vi "Unit Test Parent Level Renamed.vi"() -> ()   [LabVIEW 2019, in "Sports Unit Tests.lvclass"]
uses:
  Sports Unit Tests.lvclass
  Classes/John Cena/John Cena.lvclass
  <vilib>/Utility/error.llb/Clear Errors.vi
  <vilib>/addons/_JKI Toolkits/Caraya/classes/Test/Define Test.vi
  <vilib>/addons/_JKI Toolkits/Caraya/classes/Assert/Assert Equal Value_Variant.vi
  <vilib>/addons/_JKI Toolkits/Caraya/classes/Assert/Assert Not Error.vi
  <userlib>/Blue Origin/BlueSerialization/BlueSerializer/BlueSerializer.lvclass
  <vilib>/addons/_JKI Toolkits/Caraya/classes/Assert/Assert.lvclass
panel:
  out "Table":string[][](table)=[["{\r  \"Class\":[\"John Cena.lvclass\",\"WWF Wrestler.lvclass\",\"Sports Player.lvclass\",\"Human.lvclass\",\"BlueSerialization.lvlib:BlueSerializable.lvclass\"],\r  \"Version\":[\"2.0.0.3\",\"2.0.0.3\",\"2.0.0.3\",\"2.0.0.3\",\"2.0.0.0\"],\r  \"BlueSerialization.lvlib:BlueSerializable.lvclass\":{\"LibVersion\":1},\r  \"Human.lvclass\":{\r    \"alive?\":true,\r    \"Age (years)\":40,\r    \"Name\":\"John Cena\",\r    \"Height (ft)\":6\r  },\r  \"Sports Player.lvclass\":{\r    \"Professional?\":true,\r    \"Earnings (dollars)\":1000000,\r    \"Sponsor\":\"Monster Energy\"\r  },\r  \"WWF Wrestler.lvclass\":{\r    \"Current champion?\":false,\r    \"# champion titles\":6,\r    \"Weight (lbs)\":250\r  },\r  \"John Cena.lvclass\":{\"Latest movie role\":\"The Marine\"}\r}", "{\r  \"Class\":[\"John Cena.lvclass\",\"WWF Wrestler.lvclass\",\"Sports Player.lvclass\",\"Human.lvclass\",\"BlueSerialization.lvlib:BlueSerializable.lvclass\"],\r  \"Version\":[\"2.0.0.3\",\"2.0.0.3\",\"2.0.0.3\",\"2.0.0.3\",\"2.0.0.0\"],\r  \"BlueSerialization.lvlib:BlueSerializable.lvclass\":{\"LibVersion\":1},\r  \"Human.lvclass\":{\r    \"alive?\":true,\r    \"Age (years)\":40,\r    \"Name\":\"John Cena\",\r    \"Height (ft)\":6\r  },\r  \"Sports Player.lvclass\":{\r    \"Professional?\":true,\r    \"Earnings (dollars)\":1000000,\r    \"Sponsor\":\"Monster Energy\"\r  },\r  \"WWF Wrestler.lvclass\":{\r    \"Current champion?\":false,\r    \"# champion titles\":6,\r    \"Weight (lbs)\":250\r  },\r  \"John Cena.lvclass\":{\"Latest movie role\":\"The Marine\"}\r}", "Status: FALSE\ncode: 0\n", "BlueJSONTextSerializer.lvlib:BlueJSONTextSerializer.lvclass"], ["Class = [\"John Cena.lvclass\", \"WWF Wrestler.lvclass\", \"Sports Player.lvclass\", \"Human.lvclass\", \"BlueSerialization.lvlib:BlueSerializable.lvclass\"]\r\nVersion = [\"2.0.0.3\", \"2.0.0.3\", \"2.0.0.3\", \"2.0.0.3\", \"2.0.0.0\"]\r\n\n[\"BlueSerialization.lvlib:BlueSerializable.lvclass\"]\nLibVersion = 1\r\n\n[\"Human.lvclass\"]\n\"alive?\" = true\r\n\"Age (years)\" = 40\r\nName = \"John Cena\"\r\n\"Height (ft)\" = 6.0\r\n\n[\"Sports Player.lvclass\"]\n\"Professional?\" = true\r\n\"Earnings (dollars)\" = 1000000.0\r\nSponsor = \"Monster Energy\"\r\n\n[\"WWF Wrestler.lvclass\"]\n\"Current champion?\" = false\r\n\"# champion titles\" = 6\r\n\"Weight (lbs)\" = 250.0\r\n\n[\"John Cena.lvclass\"]\n\"Latest movie role\" = \"The Marine\"\r\n", "Class = [\"John Cena.lvclass\", \"WWF Wrestler.lvclass\", \"Sports Player.lvclass\", \"Human.lvclass\", \"BlueSerialization.lvlib:BlueSerializable.lvclass\"]\r\nVersion = [\"2.0.0.3\", \"2.0.0.3\", \"2.0.0.3\", \"2.0.0.3\", \"2.0.0.0\"]\r\n\n[\"BlueSerialization.lvlib:BlueSerializable.lvclass\"]\nLibVersion = 1\r\n\n[\"Human.lvclass\"]\n\"alive?\" = true\r\n\"Age (years)\" = 40\r\nName = \"John Cena\"\r\n\"Height (ft)\" = 6.0\r\n\n[\"Sports Player.lvclass\"]\n\"Professional?\" = true\r\n\"Earnings (dollars)\" = 1000000.0\r\nSponsor = \"Monster Energy\"\r\n\n[\"WWF Wrestler.lvclass\"]\n\"Current champion?\" = false\r\n\"# champion titles\" = 6\r\n\"Weight (lbs)\" = 250.0\r\n\n[\"John Cena.lvclass\"]\n\"Latest movie role\" = \"The Marine\"\r\n", "Status: FALSE\ncode: 0\n", "BlueTOMLSerializer.lvlib:BlueTOMLSerializer.lvclass"]]
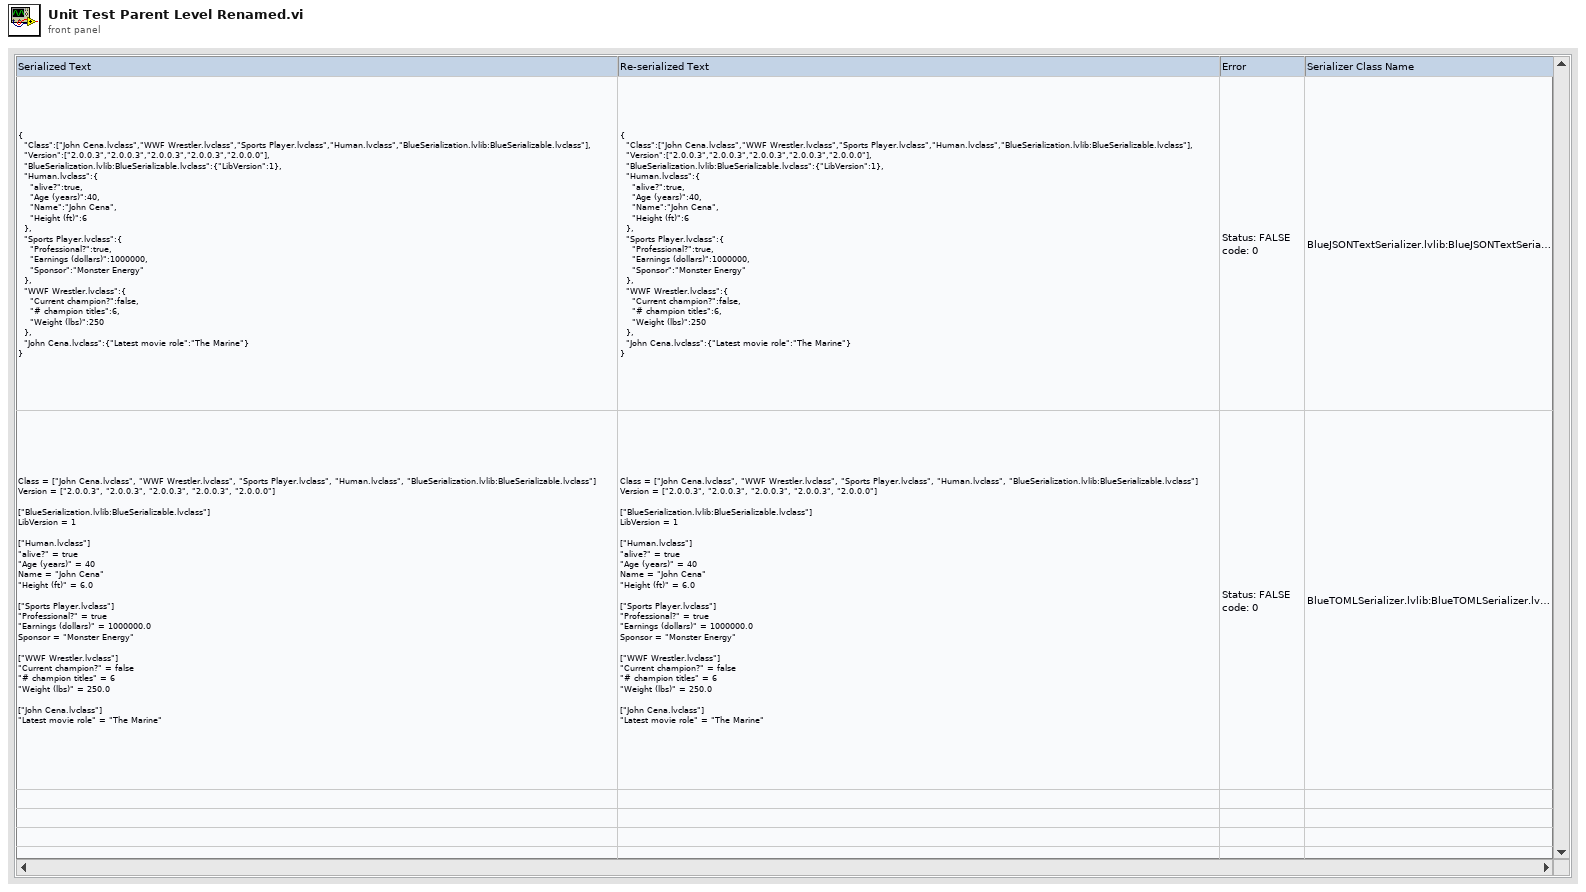
[diagram p1: front panel]
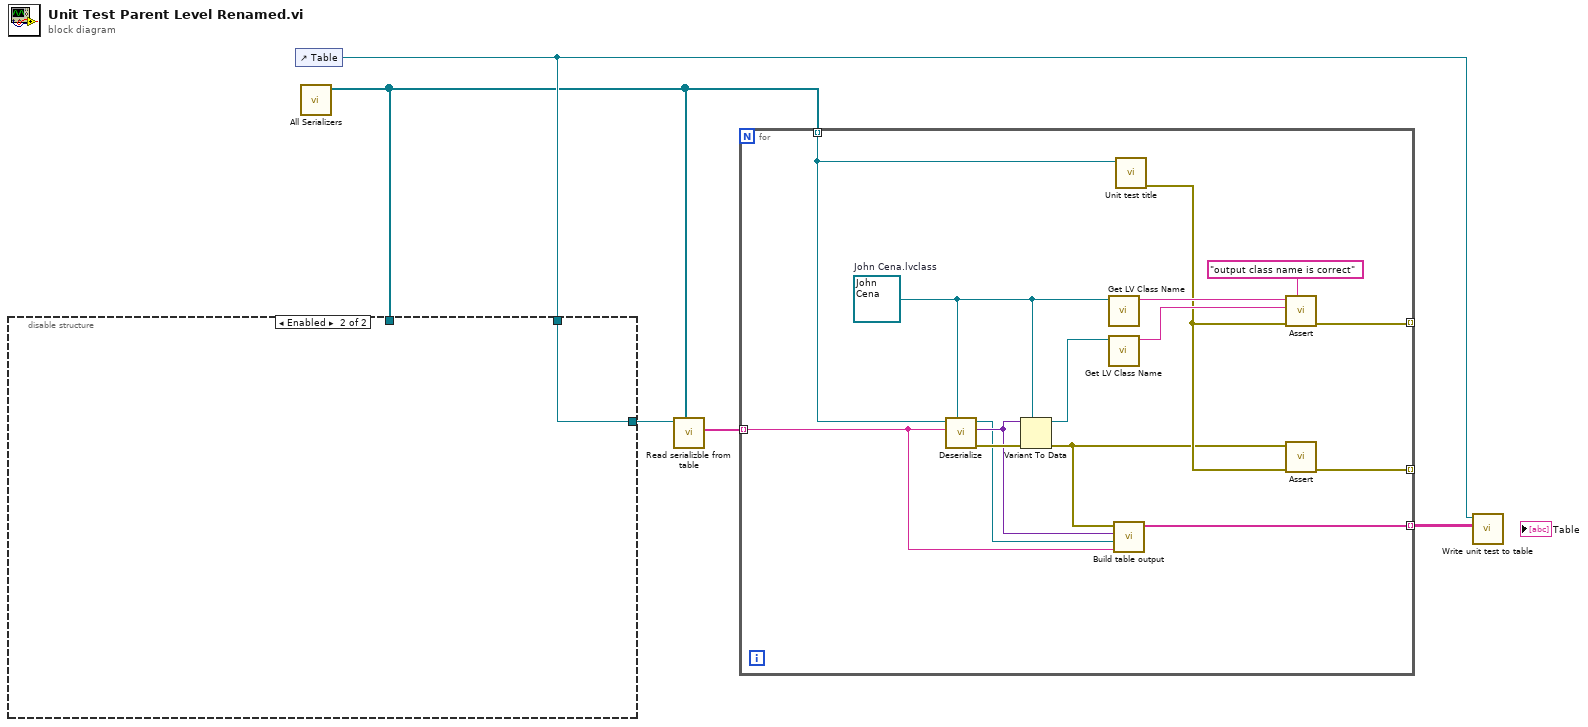
[diagram p0: block diagram]
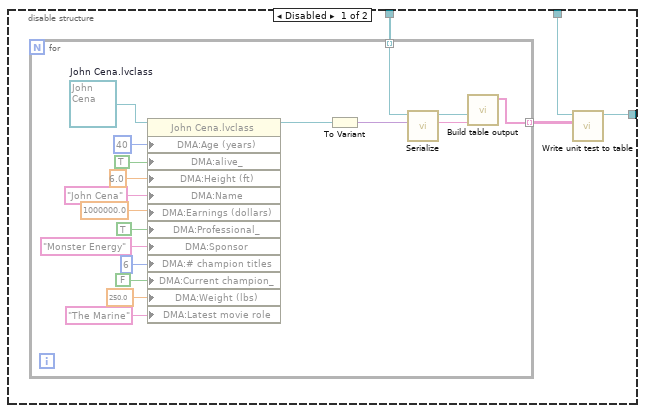
[diagram p2: hidden frame]
diagram:
  n1 = control-ref of="Table"() -> (w5:refnum<vi>)
  n2 = call "All Serializers.vi"() -> ("All serializers"=w2:refnum<class "BlueSerializer.lvclass">[])  [unwired: 11 in]
  n3 = disable-structure shown="Enabled" {
    disable-tunnel: w5 -> [w8 w28]
    disable-tunnel: [w7 w28] -> w4
    disable-tunnel: w2 -> [w6 _]
    frame Disabled {
      n4 = for {
        tunnel: w6 -> [w18] mode=indexing
        tunnel: [w15] -> w9 mode=indexing
        w14 = refnum<class "John Cena.lvclass"> refnum  # John Cena.lvclass
        n5 = property on="Property Node" class="John Cena.lvclass"(reference=w14, "DMA:Age (years)"=u16 40 ("Age (years)"), "DMA:alive_"=TRUE ("alive_"), "DMA:Height (ft)"=6.0 ("Height (ft)"), "DMA:Name"="John Cena" ("Name"), "DMA:Earnings (dollars)"=1000000.0 ("Earnings (dollars)"), "DMA:Professional_"=TRUE ("Professional_"), "DMA:Sponsor"="Monster Energy" ("Sponsor"), "DMA:# champion titles"=u8 6 ("# champion titles"), "DMA:Current champion_"=FALSE ("Current champion_"), "DMA:Weight (lbs)"=250.0 ("Weight (lbs)"), "DMA:Latest movie role"="The Marine" ("Latest movie role")) -> (reference out=w27:refnum<class "John Cena.lvclass">)  [unwired: 1 in, 1 out]
        n6 = To Variant(anything=w27) -> (Variant=w19:variant)
        n7 = call-dynamic "Serialize.vi"("Anything"=w19, "BlueSerializer in"=w18) -> ("Serialized Data"=w17:string, "BlueSerializer out"=w16:refnum<class "BlueSerializer.lvclass">)  [unwired: 7 in, 1 out]
        n8 = call "Build table output.vi"("serialized text"=w17, "BlueSerializer in"=w16) -> ("table output"=w15:string[])  [unwired: 9 in]
      }
      n9 = call "Write unit test to table.vi"("Table"=w9, "Table ref in"=w8) -> ("Table ref out"=w7:refnum<vi>)  [unwired: 9 in]
    }
    frame Enabled {
    }
  }
  n10 = call "Read serializble from table.vi"("serializers"=w2, "Table ref in"=w4) -> ("serializable texts"=w3:string[])  [unwired: 7 in, 2 out]
  n11 = for {
    tunnel: w2 -> [w30] mode=indexing
    tunnel: [w38] -> _ mode=indexing
    tunnel: [w37] -> _ mode=indexing
    tunnel: w3 -> [w32] mode=indexing
    tunnel: [w31] -> w1 mode=indexing
    w29 = refnum<class "John Cena.lvclass"> refnum  # John Cena.lvclass
    n12 = call-dynamic "Deserialize.vi"("Anything"=w29, "Serialized Object String"=w32, "BlueSerializer in"=w30) -> ("error out"=w43:errorcluster, "Variant"=w34:variant, "BlueSerializer out"=w33:refnum<class "BlueSerializer.lvclass">)  [unwired: 6 in]
    n13 = Variant To Data(error in=w43, type=w29, Variant=w34) -> (data=w42:refnum<class "John Cena.lvclass">, error out=w35:errorcluster)
    n14 = call <vilib>:"Get LV Class Name.vi"("object"=w29) -> ("class name"=w41:string)  [unwired: 9 in, 1 out]
    n15 = call <vilib>:"Get LV Class Name.vi"("object"=w42) -> ("class name"=w40:string)  [unwired: 9 in, 1 out]
    n16 = call "Build table output.vi"("serialized text"=w32, "BlueSerializer in"=w33, "deserialized variant"=w34, "variant to data error"=w35) -> ("table output"=w31:string[])  [unwired: 7 in]
    n17 = call "Unit test title.vi"("serializer"=w30) -> ("error out"=w36:errorcluster)  [unwired: 9 in, 1 out]
    n18 = call-poly <vilib>:"Assert.vi"("Label"="output class name is correct", "error in (no error)"=w36, "Y"=w40, "X"=w41) -> ("error out"=w37:errorcluster)  [unwired: 7 in]
    n19 = call-poly <vilib>:"Assert.vi"("error in (no error)"=w36, "Not Error?"=w35) -> ("error out"=w38:errorcluster)  [unwired: 9 in]
  }
  n20 = call "Write unit test to table.vi"("Table"=w1, "Table ref in"=w5) -> ()  [unwired: 9 in, 1 out]
